vi "stop_error_handling.vi"(5 "queue error in":errorcluster, 6 "state in":T1, 7 "elements in queue":T1[](array[typedef]), 8 "image error in":errorcluster, 9 "camera error in":errorcluster) -> (0 "image error out":errorcluster, 1 "camera error out":errorcluster, 2 "queue error out":errorcluster, 4 "state out":T1)   [LabVIEW 2014]
uses:
  type definitions/state machine enum.ctl
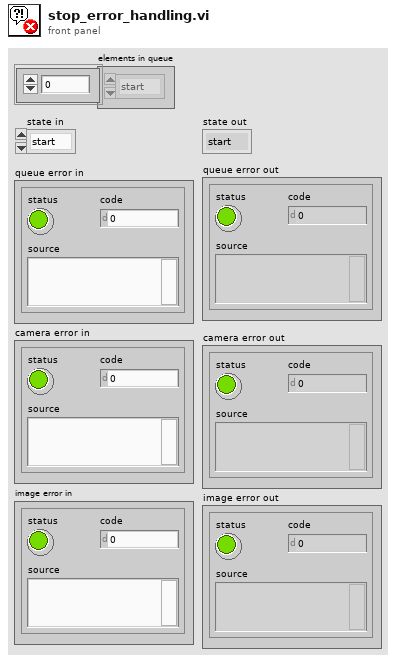
[diagram p1: front panel]
types:
  T1 = typedef "state machine enum.ctl" = enum16{"start", "select camera", "control camera properties", "calibration", "wait", "snap", "save", "save as", "grab", "error", "stop"}
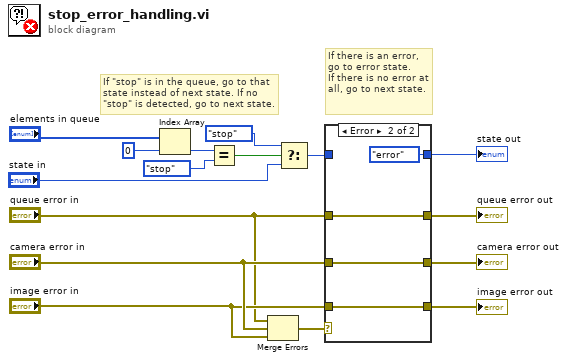
[diagram p0: block diagram]
diagram:
  # "If there is an error, go to error state. \nIf there is no error at all, go to next state."
  # "If \"stop\" is in the queue, go to that \nstate instead of next state. If no\n\"stop\" is detected, go to next state."
  n1 = Index Array(array="elements in queue", index=0) -> (element=w11:T1)
  n2 = Equal?(x=w11, y=state_machine_enum."stop" ("Zustände")) -> (x = y?=w16:bool)
  n3 = Merge Errors("queue error in", "camera error in", "image error in") -> (w10:errorcluster)
  n4 = Select(t=state_machine_enum."stop" ("Zustände"), s=w16, f="state in") -> (s? t:f=w1:T1)
  n5 = case shown="Error" w10 {
    tunnel: w1 -> [w20 _]
    tunnel: [w20 state_machine_enum."error" ("Zustände")] -> w9
    tunnel: "queue error in" -> [w19 w24]
    tunnel: [w19 w24] -> w8
    tunnel: "camera error in" -> [w17 w22]
    tunnel: "image error in" -> [w18 w21]
    tunnel: [w18 w21] -> w6
    tunnel: [w17 w22] -> w7
    frame No Error {
    }
    frame Error {
    }
  }
  "state out" <- w9
  "queue error out" <- w8
  "camera error out" <- w7
  "image error out" <- w6
